vi "ex2.vi"() -> ()   [LabVIEW 2022 SP3]
uses:
  <vilib>/numeric/Random Number (Range) I64.vi
  <vilib>/numeric/sub_Random U32.vi
panel:
  out "Array":i64[](array[numeric])
  in  "Beggining?":bool
  in  "stop":bool
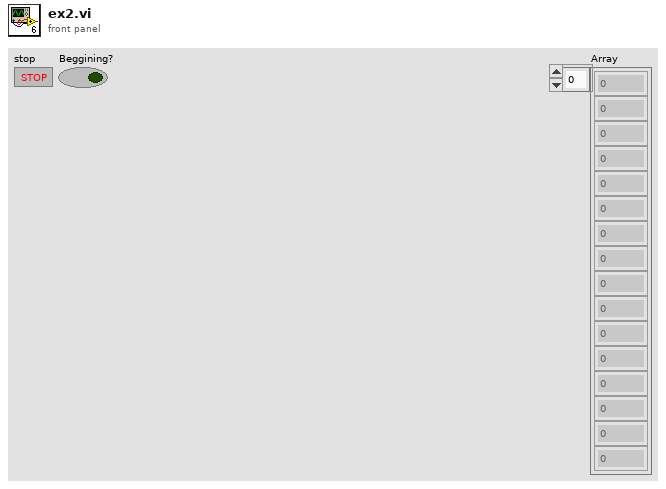
[diagram p1: front panel]
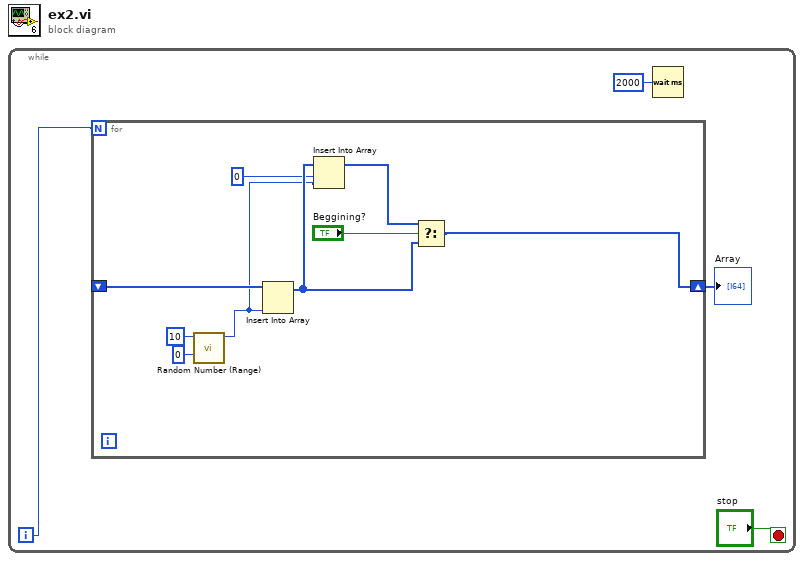
[diagram p0: block diagram]
diagram:
  n1 = while {
    i -> [w3]
    stop <- "stop" stop-if-true
    n2 = for {
      N: w3 -> [_]
      shift-right: [w8] -> w1
      shift-left: _ -> [w13]
      n3 = call-poly <vilib>:"Random Number (Range).vi"("lower bound (-100)"=i64 0, "upper bound (100)"=i64 10) -> ("number"=w5:i64)  [unwired: 9 in]
      n4 = Insert Into Array(array=w13, new element=w5) -> (w7:i64[])  [unwired: 1 in]
      n5 = Insert Into Array(array=w7, index=0, new element=w5) -> (w9:i64[])
      n6 = Select(t=w9, s="Beggining?", f=w7) -> (s? t:f=w8:i64[])
    }
    "Array" <- w1
    n7 = Wait (ms)(milliseconds to wait=u32 2000) -> ()  [unwired: 1 out]
  }
